vi "myYield2.vi"() -> (4 "Results Cluster":T1, 6 "error out":errorcluster)   [LabVIEW 2018]
uses:
  <vilib>/addons/Tools/Unicode/UTF8 Tools.lvlib
panel:
  out "Consecutive Fails":dbl
  in  "error in (no error)":errorcluster
  out "Return Code":i64
  out "Python Output":string
  in  "Path of Log":path
  out "Fails":dbl
  out "Passes":dbl
  out "Tests":dbl
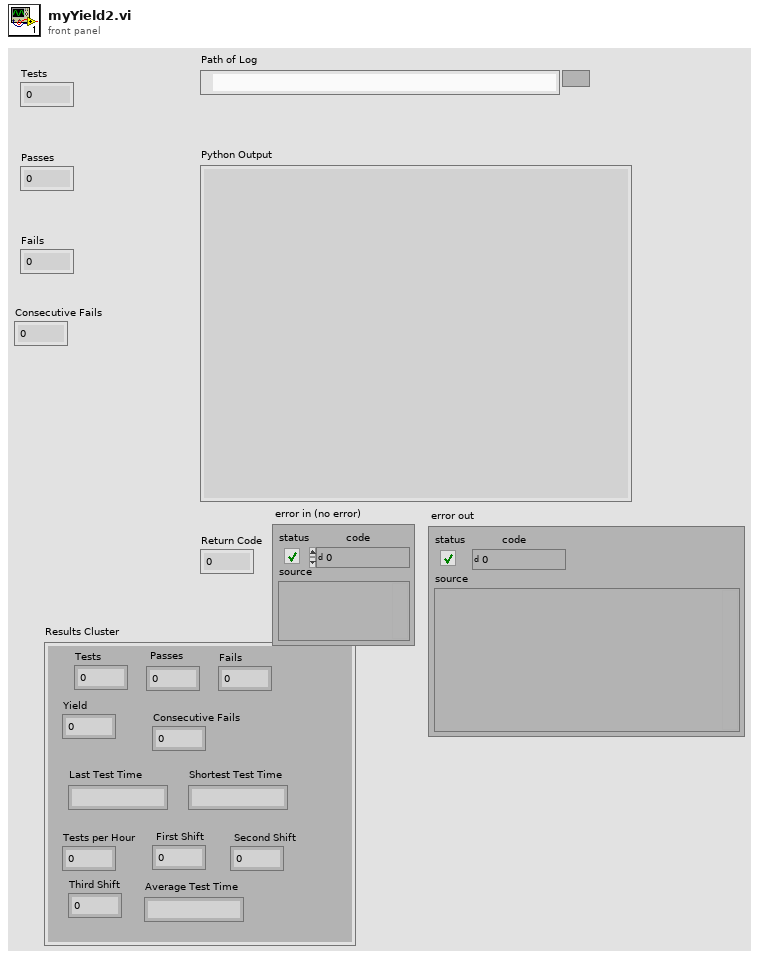
[diagram p1: front panel]
types:
  T1 = cluster{"Tests":i32, "Passes":i32, "Fails":i32, "Consecutive Fails":i32, "Yield":i32, "Last Test Time":string, "Shortest Test Time":string, "Tests per Hour":i32, " First Shift":i32, " Second Shift":i32, "Third Shift ":i32, "Average Test Time":string}
  T2 = cluster{"Tests":i32, "Passes":i32, "Fails":i32, "Consecutive Fails":i32, "Yield":i32, "Last Test Time":string, "Shortest Test Time":string, "Tests per Hour":i32, "First Shift":i32, "Second Shift":i32, "Third Shift":i32, "Average Test Time":string}
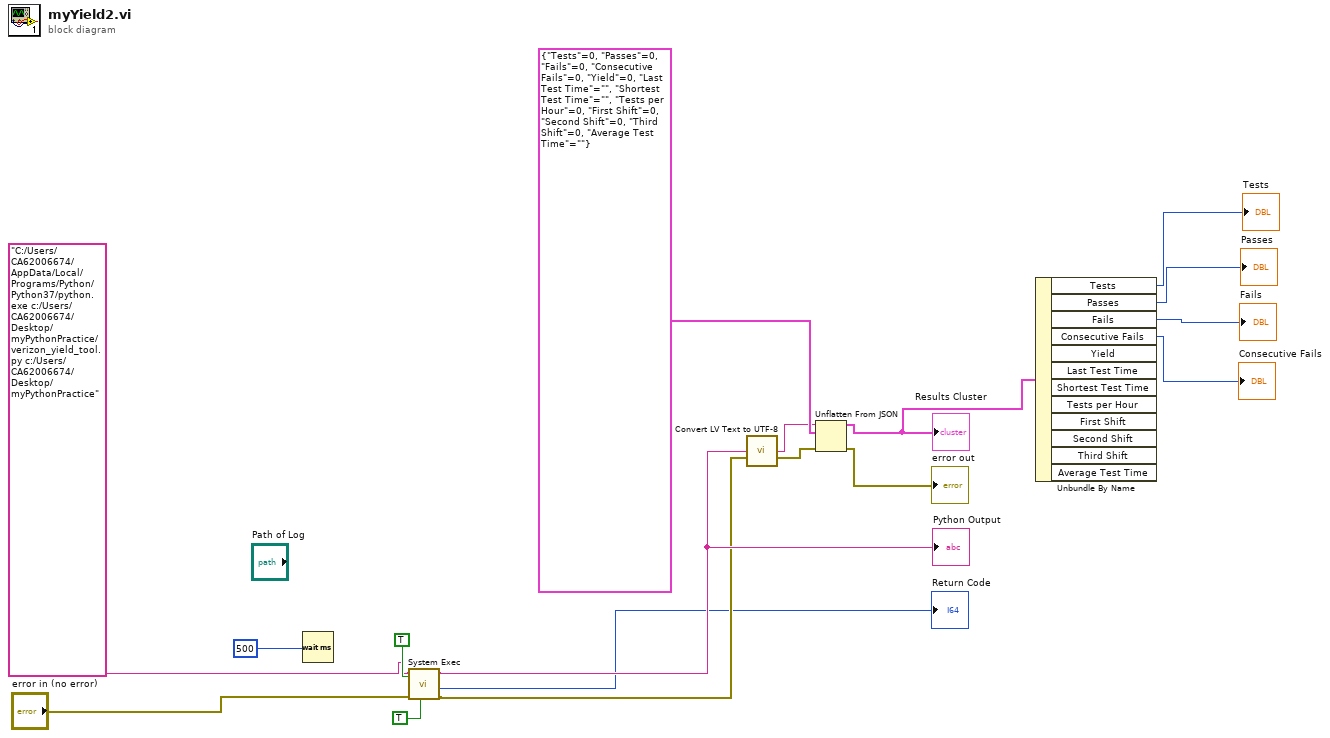
[diagram p0: block diagram]
diagram:
  n1 = Wait (ms)(milliseconds to wait=500) -> ()  [unwired: 1 out]
  n2 = call <vilib>:"System Exec.vi"("run minimized? (F)"=TRUE, "wait until completion? (T)"=TRUE, "error in (no error)"="error in (no error)", "command line"="C:/Users/CA62006674/AppData/Local/Programs/Python/Python37/python.exe c:/Users/CA62006674/Desktop/myPythonPractice/verizon_yield_tool.py c:/Users/CA62006674/Desktop/myPythonPractice") -> ("error out"=w2:errorcluster, "return code"=→"Return Code":i32, "standard output"=w3:string)  [unwired: 4 in, 1 out]
  "Python Output" <- w3
  n3 = call <vilib>:"Convert LV Text to UTF-8.vi"("LV Text"=w3, "error in"=w2) -> ("UTF-8 Text"=w16:string, "error out"=w15:errorcluster)  [unwired: 12 in]
  n4 = Unflatten From JSON(JSON string=w16, type and defaults=T2 {"Tests"=0, "Passes"=0, "Fails"=0, "Consecutive Fails"=0, "Yield"=0, "Last Test Time"="", "Shortest Test Time"="", "Tests per Hour"=0, "First Shift"=0, "Second Shift"=0, "Third Shift"=0, "Average Test Time"=""}, error in (no error)=w15) -> (value=w13:T2, error out=→"error out":errorcluster)  [unwired: 4 in]
  "Results Cluster" <- w13
  n5 = Unbundle By Name(w13) -> ("Tests"=→"Tests":i32, "Passes"=→"Passes":i32, "Fails"=→"Fails":i32, "Consecutive Fails"=→"Consecutive Fails":i32)  [unwired: 8 out]
